vi "svx_Oct_Fit Data to Scale.vi"(9 "Cropped Info":cluster{"First Index":i32, "Length":i32}, 10 "Display State In":T1={"X Scale Width %"=50.0, "Y Scale Height %"=50.0, "X-Axis Range"={"Minimum"=0.0, "Maximum"=10.0}, "Y-Axis Range"={"Minimum"=0.0, "Maximum"=10.0}, "Z-Axis Range"={"Minimum"=0.0, "Maximum"=10.0}, "Plot Color"=0, "Frame Color"=61212, "Background Color"=16252785, "Initial AutoScale Y"=TRUE, "AutoScale X"=2, "AutoScale Y"=2, "AutoScale Z"=2, "Plot Transparency"=FALSE, "X-Axis Name"="Frequency", "Y-Axis Name"="Amplitude", "Z-Axis Name"="", "X-Axis Scaling Factor"={"Offset"=0.0, "Multiplier"=1.0}, "Y-Axis Scaling Factor"={"Offset"=0.0, "Multiplier"=1.0}, "Z-Axis Scaling Factor"={"Offset"=0.0, "Multiplier"=1.0}, "X-Scale Visible"=TRUE, "Y-Scale Visible"=TRUE, "Z-Scale Visible"=TRUE, "X-Scale Label Visible"=TRUE, "Y-Scale Label Visible"=TRUE, "Z-Scale Label Visible"=TRUE, "X-Axis Range Scaled"={"Minimum"=0.0, "Maximum"=10.0}, "Y-Axis Range Scaled"={"Minimum"=0.0, "Maximum"=10.0}, "Z-Axis Range Scaled"={"Minimum"=0.0, "Maximum"=10.0}, "Rev Z Order"=FALSE, "X-Scale Format Str"="%#.4g", "Y-Scale Format Str"="%#.4g", "Z-Scale Format Str"="%#.4g", "Decor color"=12369084, "Scale Range Change"=refnum, "out of state queue"=refnum, "property nodes"=refnum} caption="State", 11 "Data In":T2={"z0"=0.0, "dz"=1.0, "Plots"=[]} {"Plots"."Y" format="%.2f"; "Plots"."X" format="%.2f"}) -> (0 "Waveform YScale Max":dbl, 1 "Waveform XScale Max":dbl, 2 "Display State Out":T1={"X Scale Width %"=50.0, "Y Scale Height %"=50.0, "X-Axis Range"={"Minimum"=0.0, "Maximum"=10.0}, "Y-Axis Range"={"Minimum"=0.0, "Maximum"=10.0}, "Z-Axis Range"={"Minimum"=0.0, "Maximum"=10.0}, "Plot Color"=0, "Frame Color"=61212, "Background Color"=16252785, "Initial AutoScale Y"=TRUE, "AutoScale X"=2, "AutoScale Y"=2, "AutoScale Z"=2, "Plot Transparency"=FALSE, "X-Axis Name"="Frequency", "Y-Axis Name"="Amplitude", "Z-Axis Name"="", "X-Axis Scaling Factor"={"Offset"=0.0, "Multiplier"=1.0}, "Y-Axis Scaling Factor"={"Offset"=0.0, "Multiplier"=1.0}, "Z-Axis Scaling Factor"={"Offset"=0.0, "Multiplier"=1.0}, "X-Scale Visible"=TRUE, "Y-Scale Visible"=TRUE, "Z-Scale Visible"=TRUE, "X-Scale Label Visible"=TRUE, "Y-Scale Label Visible"=TRUE, "Z-Scale Label Visible"=TRUE, "X-Axis Range Scaled"={"Minimum"=0.0, "Maximum"=10.0}, "Y-Axis Range Scaled"={"Minimum"=0.0, "Maximum"=10.0}, "Z-Axis Range Scaled"={"Minimum"=0.0, "Maximum"=10.0}, "Rev Z Order"=FALSE, "X-Scale Format Str"="%#.4g", "Y-Scale Format Str"="%#.4g", "Z-Scale Format Str"="%#.4g", "Decor color"=12369084, "Scale Range Change"=refnum, "out of state queue"=refnum, "property nodes"=refnum} caption="State", 3 "Data Out":T2={"z0"=0.0, "dz"=1.0, "Plots"=[]} {"Plots"."Y" format="%.2f"; "Plots"."X" format="%.2f"}, 4 "Markers":dbl[](array[numeric]))   [LabVIEW 2017, in "SVX Octave Waterfall Graph.xctl"]
uses:
  <vilib>/addons/_XControls/Octave Waterfall Graph/SVX Octave Waterfall Graph.xctl
  <vilib>/addons/_XControls/Octave Waterfall Graph/subVIs/svx_Oct_Waterfall Data.ctl
  <vilib>/addons/_XControls/Octave Waterfall Graph/subVIs/svx_Oct_Waterfall State.ctl
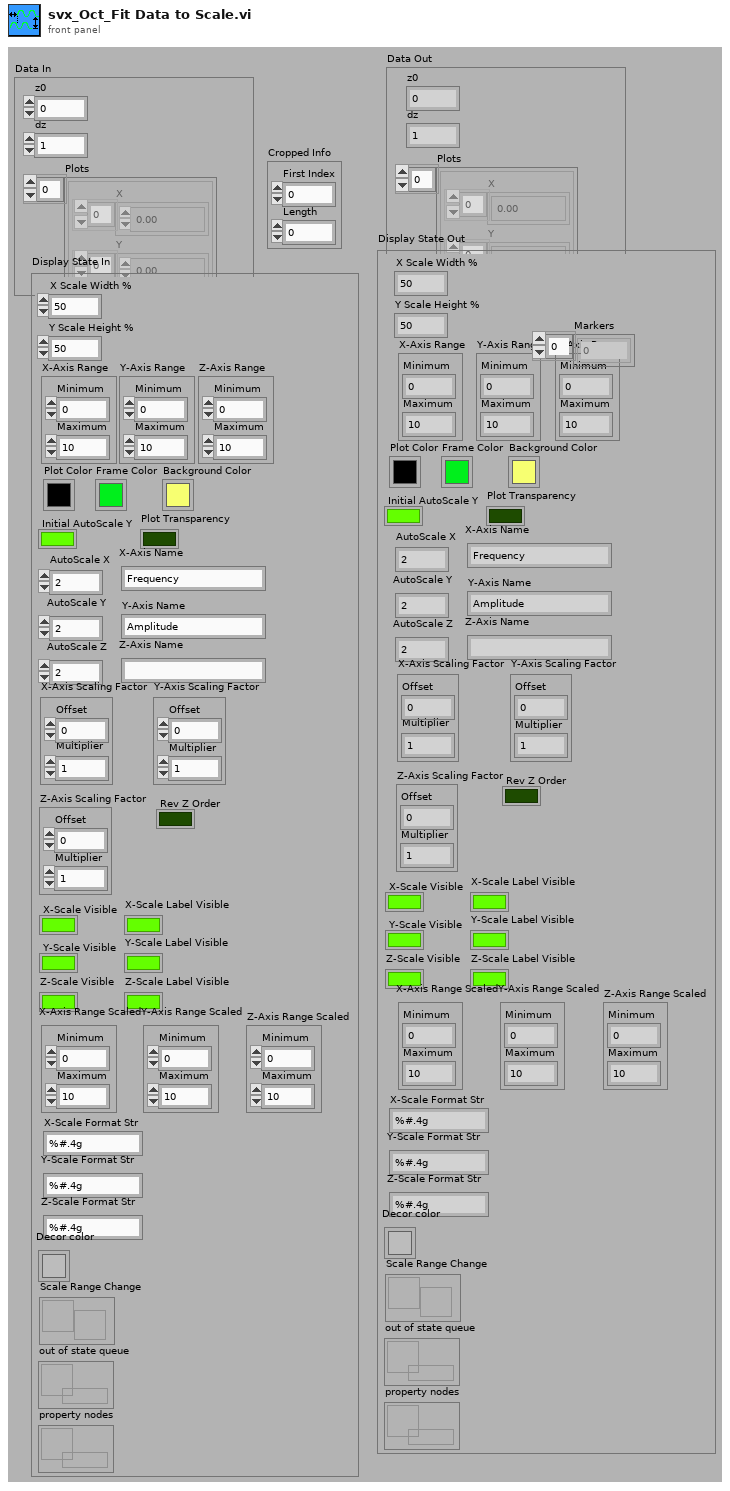
[diagram p1: front panel]
types:
  T1 = typedef "SVX Octave Waterfall Graph.xctl/svx_Oct_Waterfall State.ctl" = cluster{"X Scale Width %":dbl, "Y Scale Height %":dbl, "X-Axis Range":cluster{"Minimum":dbl, "Maximum":dbl}, "Y-Axis Range":cluster{"Minimum":dbl, "Maximum":dbl}, "Z-Axis Range":cluster{"Minimum":dbl, "Maximum":dbl}, "Plot Color":u32, "Frame Color":u32, "Background Color":u32, "Initial AutoScale Y":bool, "AutoScale X":u8, "AutoScale Y":u8, "AutoScale Z":u8, "Plot Transparency":bool, "X-Axis Name":string, "Y-Axis Name":string, "Z-Axis Name":string, "X-Axis Scaling Factor":cluster{"Offset":dbl, "Multiplier":dbl}, "Y-Axis Scaling Factor":cluster{"Offset":dbl, "Multiplier":dbl}, "Z-Axis Scaling Factor":cluster{"Offset":dbl, "Multiplier":dbl}, "X-Scale Visible":bool, "Y-Scale Visible":bool, "Z-Scale Visible":bool, "X-Scale Label Visible":bool, "Y-Scale Label Visible":bool, "Z-Scale Label Visible":bool, "X-Axis Range Scaled":cluster{"Minimum":dbl, "Maximum":dbl}, "Y-Axis Range Scaled":cluster{"Minimum":dbl, "Maximum":dbl}, "Z-Axis Range Scaled":cluster{"Minimum":dbl, "Maximum":dbl}, "Rev Z Order":bool, "X-Scale Format Str":string, "Y-Scale Format Str":string, "Z-Scale Format Str":string, "Decor color":u32, "Scale Range Change":refnum<user-event>, "out of state queue":refnum<queue>, "property nodes":refnum<queue>}
  T2 = typedef "SVX Octave Waterfall Graph.xctl/svx_Oct_Waterfall Data.ctl" = cluster{"z0":dbl, "dz":dbl, "Plots":cluster{"X":dbl[], "Y":dbl[]}[]}
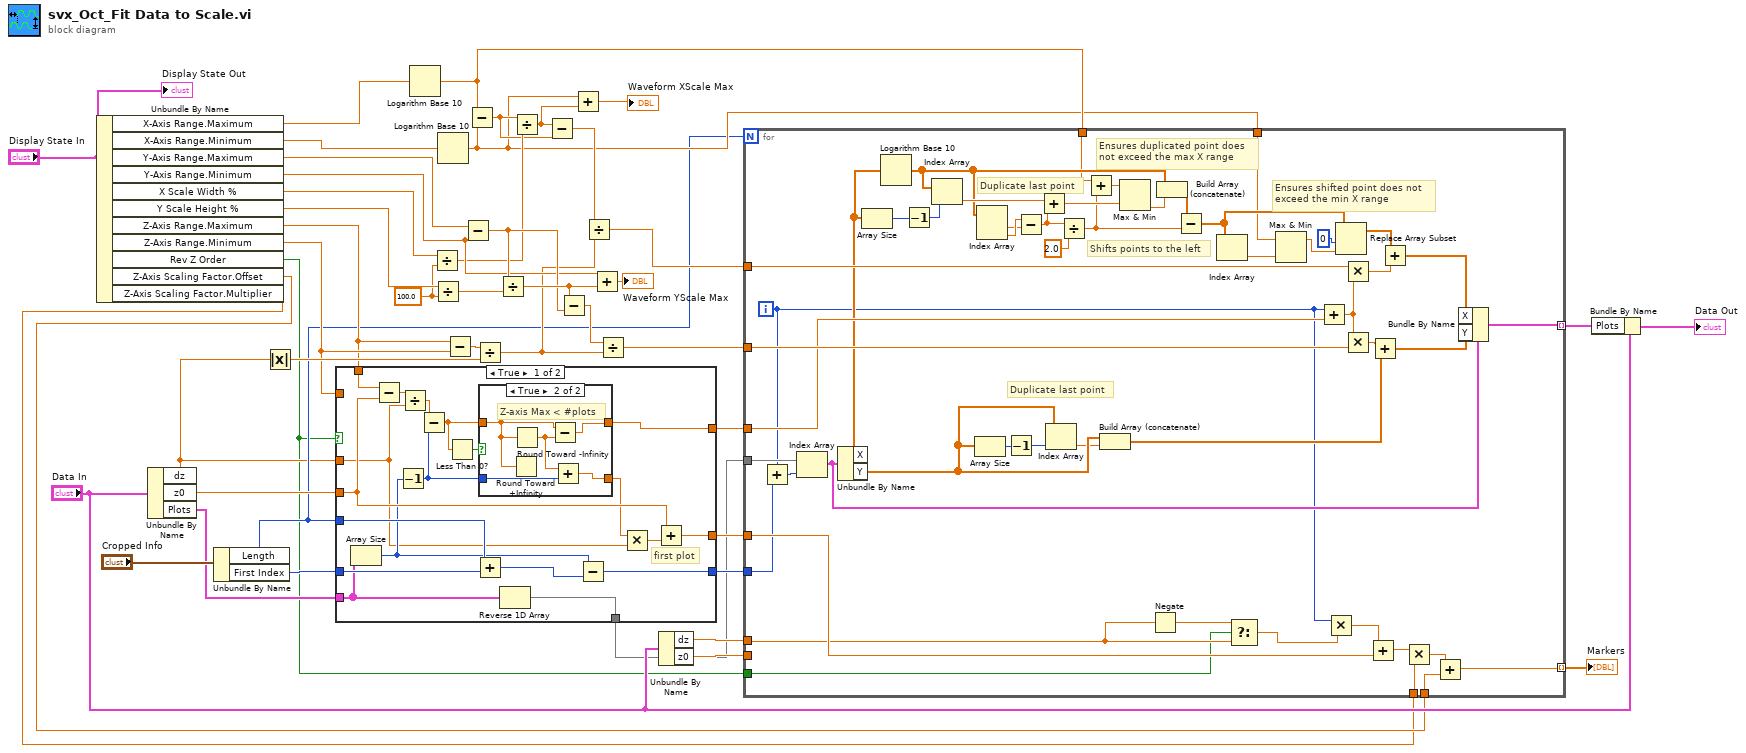
[diagram p0: block diagram]
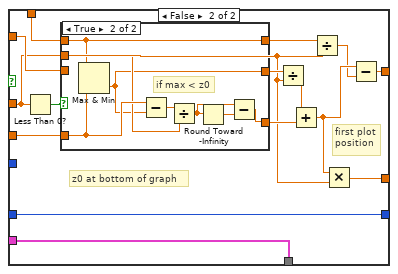
[diagram p3: hidden frame]
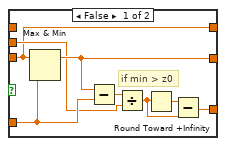
[diagram p4: hidden frame]
diagram:
  w34 = 100.0 ("y")
  n1 = Unbundle By Name("Display State In") -> ("X-Axis Range.Maximum"=w12:dbl, "X-Axis Range.Minimum"=w10:dbl, "Y-Axis Range.Maximum"=w41:dbl, "Y-Axis Range.Minimum"=w40:dbl, "X Scale Width %"=w35:dbl, "Y Scale Height %"=w37:dbl, "Z-Axis Range.Maximum"=w28:dbl, "Z-Axis Range.Minimum"=w29:dbl, "Rev Z Order"=w1:bool, "Z-Axis Scaling Factor.Offset"=w21:dbl, "Z-Axis Scaling Factor.Multiplier"=w20:dbl)
  n2 = Unbundle By Name("Data In") -> ("dz"=w2:dbl, "z0"=w31:dbl, "Plots"=w4:cluster{"X":dbl[], "Y":dbl[]}[])
  n3 = Unbundle By Name("Cropped Info") -> ("Length"=w7:i32, "First Index"=w6:i32)
  n4 = Absolute Value(x=w2) -> (abs(x)=w30:dbl)
  n5 = case shown="True" w1 {
    tunnel: [w50 w87] -> w38
    tunnel: w31 -> [w60 w84]
    tunnel: w29 -> [_ w86]
    tunnel: w28 -> [w61 w85]
    tunnel: w2 -> [w47 w73]
    tunnel: [w59 w79] -> w22
    tunnel: w7 -> [w55 _]
    tunnel: [w58 w76] -> w5
    tunnel: w6 -> [w56 w76]
    tunnel: w4 -> [w54 w75]
    tunnel: [w57 w75] -> w3
    frame True {
      # "first plot"
      n6 = Array Size(array=w54) -> (size(s)=w53:i32)
      n7 = Subtract(x=w61, y=w60) -> (x-y=w63:dbl)
      n8 = Decrement(x=w53) -> (x-1=w49:i32)
      n9 = Divide(x=w63, y=w47) -> (x/y=w65:dbl)
      n10 = Subtract(x=w65, y=w49) -> (x-y=w51:dbl)
      n11 = Less Than 0?(x=w51) -> (x < 0?=w52:bool)
      n12 = Add(x=w55, y=w56) -> (x+y=w62:i32)
      n13 = case shown="True" w52 {
        tunnel: w51 -> [w67 w71]
        tunnel: [w67 w72] -> w50
        tunnel: [w66 w69] -> w48
        tunnel: w49 -> [w66 w70]
        frame False {
          # "Z-axis Max > #plots"
        }
        frame True {
          # "Z-axis Max < #plots"
          n14 = Round Toward +Infinity(x=w71) -> ()  [unwired: 1 out]
          n15 = Round Toward -Infinity(1:w71) -> (0:w68:dbl)
          n16 = Subtract(x=w71, y=w68) -> (x-y=w72:dbl)
          n17 = Add(x=w68, y=w70) -> (x+y=w69:dbl)
        }
      }
      n18 = Reverse 1D Array(array=w54) -> (reversed array=w57:cluster{"X":dbl[], "Y":dbl[]}[])
      n19 = Subtract(x=w53, y=w62) -> (x-y=w58:i32)
      n20 = Multiply(x=w48, y=w47) -> (x*y=w64:dbl)
      n21 = Add(x=w60, y=w64) -> (x+y=w59:dbl)
    }
    frame False {
      # "first plot\nposition"
      # "z0 at bottom of graph"
      n22 = Less Than 0?(x=w73) -> (x < 0?=w74:bool)
      n23 = case shown="True" w74 {
        tunnel: w86 -> [w88 _]
        tunnel: w85 -> [_ w96]
        tunnel: w84 -> [w95 w103]
        tunnel: [w88 w96] -> w83
        tunnel: [w94 w97] -> w82
        tunnel: [w90 w100] -> w81
        tunnel: w73 -> [w89 w101]
        frame False {
          # "if min > z0"
          n24 = Max & Min(x=w88, y=w95) -> (max(x,y)=w90:dbl)  [unwired: 1 out]
          n25 = Subtract(x=w90, y=w95) -> (x-y=w93:dbl)
          n26 = Divide(x=w93, y=w89) -> (x/y=w91:dbl)
          n27 = Round Toward +Infinity(x=w91) -> (ceil(x): smallest int >= x=w92:dbl)
          n28 = Subtract(x=w92, y=w91) -> (x-y=w94:dbl)
        }
        frame True {
          # "if max < z0"
          n29 = Max & Min(x=w96, y=w103) -> (min(x,y)=w100:dbl)  [unwired: 1 out]
          n30 = Subtract(x=w103, y=w100) -> (x-y=w102:dbl)
          n31 = Divide(x=w102, y=w101) -> (x/y=w98:dbl)
          n32 = Round Toward -Infinity(1:w98) -> (0:w99:dbl)
          n33 = Subtract(x=w98, y=w99) -> (x-y=w97:dbl)
        }
      }
      n34 = Divide(x=w81, y=w73) -> (x/y=w80:dbl)
      n35 = Add(x=w80, y=w82) -> (x+y=w78:dbl)
      n36 = Divide(x=w83, y=w73) -> (x/y=w77:dbl)
      n37 = Multiply(x=w78, y=w73) -> (x*y=w79:dbl)
      n38 = Subtract(x=w78, y=w77) -> (x-y=w87:dbl)
    }
  }
  n39 = Logarithm Base 10(1:w12) -> (0:w11:dbl)
  n40 = Divide(x=w35, y=w34) -> (x/y=w19:dbl)
  n41 = Divide(x=w37, y=w34) -> (x/y=w36:dbl)
  n42 = Logarithm Base 10(1:w10) -> (0:w9:dbl)
  n43 = Subtract(x=w28, y=w29) -> (x-y=w39:dbl)
  n44 = Subtract(x=w41, y=w40) -> (x-y=w44:dbl)
  n45 = Subtract(x=w11, y=w9) -> (x-y=w15:dbl)
  n46 = Divide(x=w39, y=w30) -> (x/y=w17:dbl)
  n47 = Divide(x=w44, y=w36) -> (x/y=w46:dbl)
  n48 = Divide(x=w15, y=w19) -> (x/y=w16:dbl)
  n49 = Subtract(x=w16, y=w15) -> (x-y=w18:dbl)
  n50 = Subtract(x=w46, y=w44) -> (x-y=w45:dbl)
  n51 = Add(x=w9, y=w16) -> (x+y=→"Waveform XScale Max":dbl)
  n52 = Divide(x=w18, y=w17) -> (x/y=w14:dbl)
  n53 = Add(x=w40, y=w46) -> (x+y=→"Waveform YScale Max":dbl)
  n54 = Divide(x=w45, y=w17) -> (x/y=w43:dbl)
  n55 = Unbundle By Name("Data In") -> ("dz"=w24:dbl, "z0"=w25:dbl)
  n56 = for {
    N: w7 -> [_]
    tunnel: w14 -> [w154]
    tunnel: [w153] -> w32 mode=indexing
    tunnel: w43 -> [w152]
    tunnel: w38 -> [w150]
    tunnel: w25 -> [_]
    tunnel: w24 -> [w106]
    tunnel: [w141] -> w23 mode=indexing
    tunnel: w22 -> [w146]
    tunnel: w21 -> [w142]
    tunnel: w20 -> [w143]
    tunnel: w11 -> [w123]
    tunnel: w9 -> [w116]
    tunnel: w3 -> [w111]
    tunnel: w5 -> [w108]
    tunnel: w1 -> [w104]
    i -> [w109]
    # "Duplicate last point"
    # "Ensures shifted point does not\nexceed the min X range"
    # "Ensures duplicated point does\nnot exceed the max X range"
    # "Duplicate last point"
    # "Shifts points to the left"
    n57 = Add(x=w109, y=w108) -> (x+y=w112:i32)
    n58 = Index Array(array=w111, index=w112) -> (element=w110:cluster{"X":dbl[], "Y":dbl[]})
    n59 = Unbundle By Name(w110) -> ("X"=w115:dbl[], "Y"=w129:dbl[])
    n60 = Array Size(array=w115) -> (size(s)=w136:i32)
    n61 = Logarithm Base 10(1:w115) -> (0:w126:dbl[])
    n62 = Decrement(x=w136) -> (x-1=w135:i32)
    n63 = Index Array(array=w126, index=w135) -> (element=w134:dbl)
    n64 = Array Size(array=w129) -> (size(s)=w130:i32)
    n65 = Index Array(array=w126) -> (element #1=w138:dbl, element #2=w139:dbl)  [unwired: 2 in]
    n66 = Decrement(x=w130) -> (x-1=w131:i32)
    n67 = Subtract(x=w139, y=w138) -> (x-y=w133:dbl)
    n68 = Add(x=w134, y=w133) -> (x+y=w125:dbl)
    n69 = Index Array(array=w129, index=w131) -> (element=w128:dbl)
    n70 = Divide(x=w133, y=2.0) -> (x/y=w121:dbl)
    n71 = Add(x=w123, y=w121) -> (x+y=w122:dbl)
    n72 = Build Array (concatenate)(w129, w128) -> (w127:dbl[])
    n73 = Max & Min(x=w122, y=w125) -> (min(x,y)=w124:dbl)  [unwired: 1 out]
    n74 = Negate(x=w106) -> (-x=w107:dbl)
    n75 = Build Array (concatenate)(w126, w124) -> (w132:dbl[])
    n76 = Subtract(x=w132, y=w121) -> (x-y=w118:dbl[])
    n77 = Index Array(array=w118) -> (element=w119:dbl)  [unwired: 1 in]
    n78 = Select(t=w107, s=w104, f=w106) -> (s? t:f=w105:dbl)
    n79 = Max & Min(x=w116, y=w119) -> (max(x,y)=w114:dbl)  [unwired: 1 out]
    n80 = Add(x=w109, y=w150) -> (x+y=w151:dbl)
    n81 = Multiply(x=w109, y=w105) -> (x*y=w147:dbl)
    n82 = Replace Array Subset(array=w118, new element=w114, index=0) -> (w117:dbl[])
    n83 = Multiply(x=w154, y=w151) -> (x*y=w140:dbl)
    n84 = Multiply(x=w151, y=w152) -> (x*y=w149:dbl)
    n85 = Add(x=w147, y=w146) -> (x+y=w144:dbl)
    n86 = Add(x=w149, y=w127) -> (x+y=w148:dbl[])
    n87 = Add(x=w117, y=w140) -> (x+y=w113:dbl[])
    n88 = Multiply(x=w144, y=w143) -> (x*y=w145:dbl)
    n89 = Add(x=w145, y=w142) -> (x+y=w141:dbl)
    n90 = Bundle By Name(cluster=w110, "X"=w113, "Y"=w148) -> (w153:cluster{"X":dbl[], "Y":dbl[]})
  }
  "Markers" <- w23
  n91 = Bundle By Name(cluster="Data In", "Plots"=w32) -> (→"Data Out":T2)
  "Display State Out" <- "Display State In"
